vi "PS_depth.vi"(4 "error in (no error)":errorcluster, 5 "Calibrate":bool, 7 "Water density [kg/m^3]":dbl=1000.0) -> (0 "error out":errorcluster, 1 "P_ref [Pa]":dbl, 2 "Pressure [Bar]":dbl, 3 "Depth [m]":dbl)   [LabVIEW 2013]
uses:
  My Computer/Controls/Advanced Swimbladder Indicators.ctl
  <vilib>/myRIO/Instrument Drivers/Onboard IO/AI/vis/Smart Open.vi
  <vilib>/myRIO/Instrument Drivers/Onboard IO/AI/vis/Read.vi
  <vilib>/myRIO/Instrument Drivers/Onboard IO/AI/vis/Open.vi
  <vilib>/myRIO/Common/Instrument Driver Framework/myRIO v1.0/AI/vis/myRIO v1.1 Open AI.vi
  <vilib>/myRIO/Common/Instrument Driver Framework/Utilities/vis/Validate Channels.vi
  <vilib>/myRIO/Common/Instrument Driver Framework/myRIO v1.0/AI/vis/myRIO v1.0 Reserve AI.vi
  <vilib>/myRIO/Common/Instrument Driver Framework/myRIO v1.0/AI/vis/myRIO v1.0 Build MUX Configuration AI.vi
  <vilib>/myRIO/Common/Instrument Driver Framework/myRIO v1.0/Resource Manager/vis/myRIO v1.0 Reserve Channel List.vi
  <vilib>/myRIO/Common/Instrument Driver Framework/myRIO v1.0/Resource Manager/vis/myRIO v1.0 Reserve Channel.vi
  <vilib>/myRIO/Common/Instrument Driver Framework/myRIO v1.0/Resource Manager/vis/myRIO v1.0 Unreserve Channel.vi
  <vilib>/myRIO/Common/Instrument Driver Framework/myRIO v1.0/Resource Manager/vis/myRIO v1.0 Build Mutex Name.vi
  <vilib>/myRIO/Common/Instrument Driver Framework/myRIO v1.0/myRIO v1.1 Open.vi
  <vilib>/myRIO/Common/Instrument Driver Framework/myRIO v1.0/AI/vis/myRIO v1.0 Get Scaling Constants AI.vi
  <vilib>/Utility/VariantDataType/GetNumericInfo.vi
  <vilib>/Utility/error.llb/Error Cluster From Error Code.vi
  <vilib>/myRIO/Common/Instrument Driver Framework/Utilities/vis/IO Manager.vi
  <vilib>/myRIO/Common/Instrument Driver Framework/Utilities/vis/Configuration Manager.vi
  <vilib>/myRIO/Common/Instrument Driver Framework/myRIO v1.0/myRIO v1.0 Close.vi
  <vilib>/myRIO/Common/Instrument Driver Framework/myRIO v1.0/AI/vis/myRIO v1.0 Read AI.vi
panel:
  out "Uout Pressure  [V]":dbl
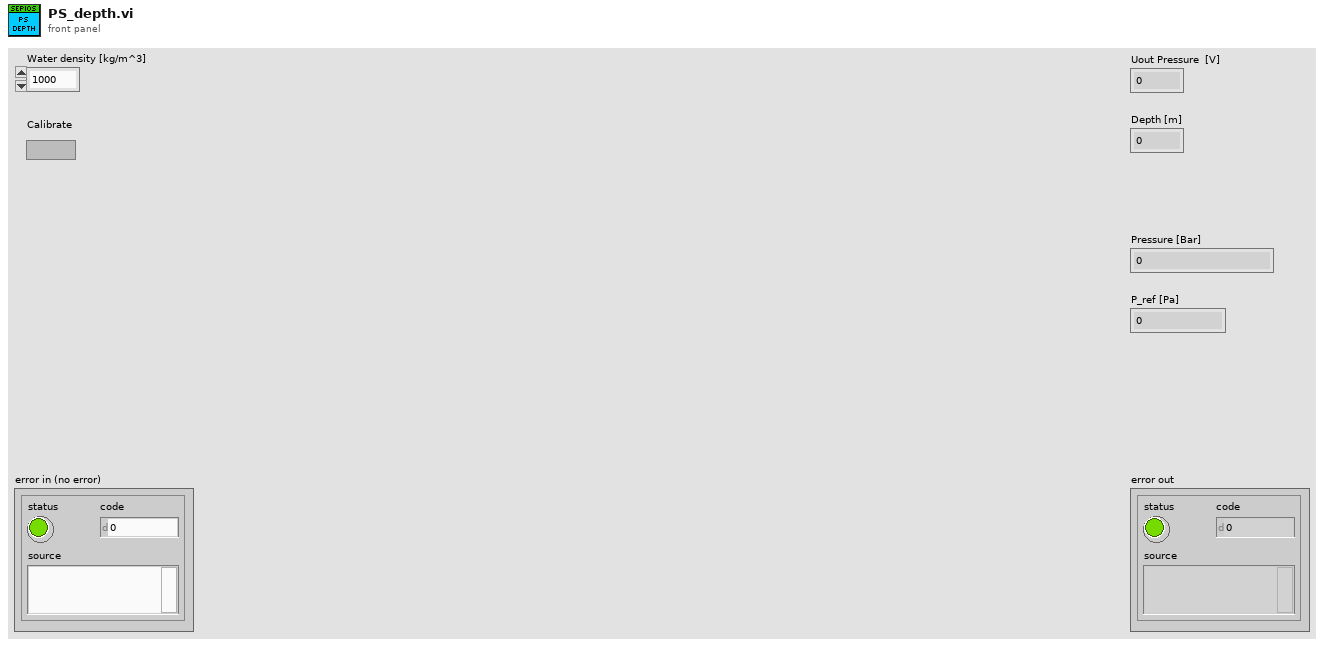
[diagram p1: front panel]
types:
  T1 = typedef "Advanced Swimbladder Indicators.ctl" = cluster{"P_ref [Pa]":dbl, "X_Actual [m]":dbl, "Motor Current[A]":dbl}
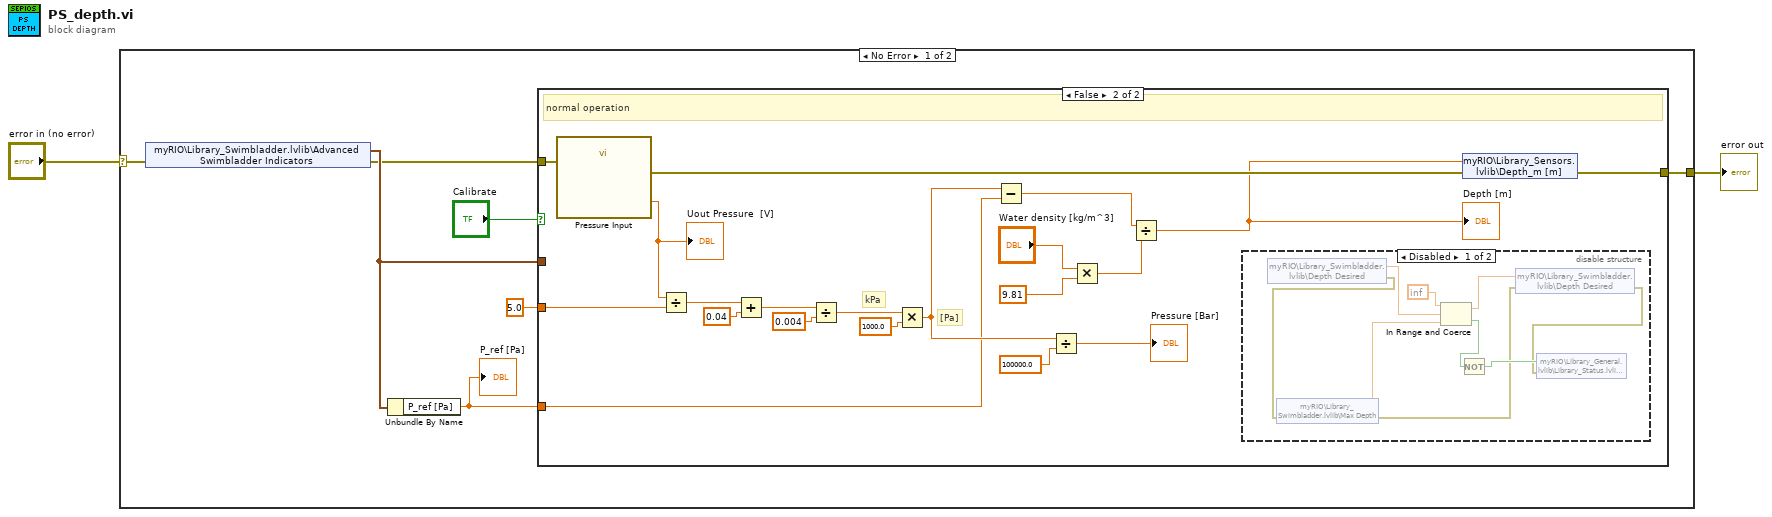
[diagram p0: block diagram]
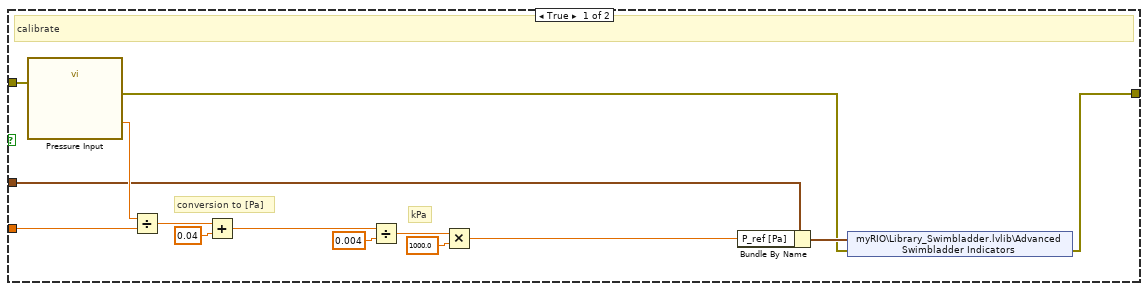
[diagram p2: hidden frame]
diagram:
  n1 = case shown="No Error" "error in (no error)" {
    selector: "error in (no error)" -> [w3 w53]
    tunnel: [w7 w53] -> w2
    frame No Error {
      n2 = shared-variable "myRIO\\Library_Swimbladder.lvlib\\Advanced Swimbladder Indicators"(error in=w3) -> (w6:T1, error out=w4:errorcluster)
      n3 = Unbundle By Name(w6) -> ("P_ref [Pa]"=w5:dbl)
      "P_ref [Pa]" <- w5
      n4 = case shown="False" "Calibrate" {
        tunnel: w4 -> [w19 w43]
        tunnel: w5 -> [_ w29]
        tunnel: [w10 w25] -> w7
        tunnel: 5.0 ("VSupply") -> [w18 w33]
        tunnel: w6 -> [w12 _]
        frame True {
          # "kPa"
          # "conversion to [Pa]"
          # "calibrate"
          n5 = call "Pressure Input"("error in (no error)"=w19) -> ("PRESSURE_SENSOR (A/AI1 (Pin 5))"=w15:dbl, "error out"=w11:errorcluster)  [unwired: 25 in]
          n6 = Divide(x=w15, y=w18) -> (x/y=w23:dbl)
          n7 = Add(x=w23, y=0.04) -> (x+y=w21:dbl)
          n8 = Divide(x=w21, y=0.004) -> (x/y=w17:dbl)
          n9 = Multiply(x=w17, y=1000.0) -> (x*y=w14:dbl)
          n10 = Bundle By Name(cluster=w12, "P_ref [Pa]"=w14) -> (w13:T1)
          n11 = shared-variable "myRIO\\Library_Swimbladder.lvlib\\Advanced Swimbladder Indicators"(w13, error in=w11) -> (error out=w10:errorcluster)
        }
        frame False {
          # "kPa"
          # "[Pa]"
          # "normal operation"
          n12 = call "Pressure Input"("error in (no error)"=w43) -> ("PRESSURE_SENSOR (A/AI1 (Pin 5))"=w35:dbl, "error out"=w26:errorcluster)  [unwired: 25 in]
          "Uout Pressure  [V]" <- w35
          n13 = Divide(x=w35, y=w33) -> (x/y=w42:dbl)
          n14 = Add(x=w42, y=0.04) -> (x+y=w40:dbl)
          n15 = Divide(x=w40, y=0.004) -> (x/y=w32:dbl)
          n16 = Multiply(x=w32, y=1000.0) -> (x*y=w30:dbl)
          n17 = Subtract(x=w30, y=w29) -> (x-y=w37:dbl)
          n18 = Divide(x=w30, y=100000.0) -> (x/y=→"Pressure [Bar]":dbl)
          n19 = Multiply(x="Water density [kg/m^3]", y=9.81) -> (x*y=w36:dbl)
          n20 = Divide(x=w37, y=w36) -> (x/y=w24:dbl)
          "Depth [m]" <- w24
          n21 = disable-structure shown="Disabled" {
            frame Disabled {
              n22 = shared-variable "myRIO\\Library_Swimbladder.lvlib\\Depth Desired"() -> (w48:dbl, error out=w46:errorcluster)  [unwired: 1 in]
              n23 = shared-variable "myRIO\\Library_Swimbladder.lvlib\\Max Depth"(error in=w46) -> (w50:dbl, error out=w45:errorcluster)
              n24 = In Range and Coerce(upper limit=inf, x=w48, lower limit=w50) -> (coerced(x)=w47:dbl, In Range?=w52:bool)
              n25 = Not(x=w52) -> (.not. x?=w51:bool)
              n26 = shared-variable "myRIO\\Library_Swimbladder.lvlib\\Depth Desired"(w47, error in=w45) -> (error out=w44:errorcluster)
              n27 = shared-variable "myRIO\\Library_General.lvlib\\Library_Status.lvlib\\tooDeep"(w51, error in=w44) -> ()  [unwired: 1 out]
            }
            frame Enabled {
            }
          }
          n28 = shared-variable "myRIO\\Library_Sensors.lvlib\\Depth_m [m]"(w24, error in=w26) -> (error out=w25:errorcluster)
        }
      }
    }
    frame Error {
    }
  }
  "error out" <- w2
